vi "Test Write Speed.vi"(8 "error in (no error)":errorcluster, 11 "Path":path) -> (0 "error out":errorcluster, 1 "sizes":T2, 2 "Write Times":T1)   [LabVIEW 2016]
uses:
  Data.ITX/Data.ITX.lvclass
  Data/Data.lvclass
  Data/Typedefs/Dictionary--cluster.ctl
  Data/Typedefs/File Type--enum.ctl
  C:/Users/patrick/Documents/GitHub/LV-to-ITX/src/Data/Data.lvclass
panel:
  out "State":string
  in  "OK":bool
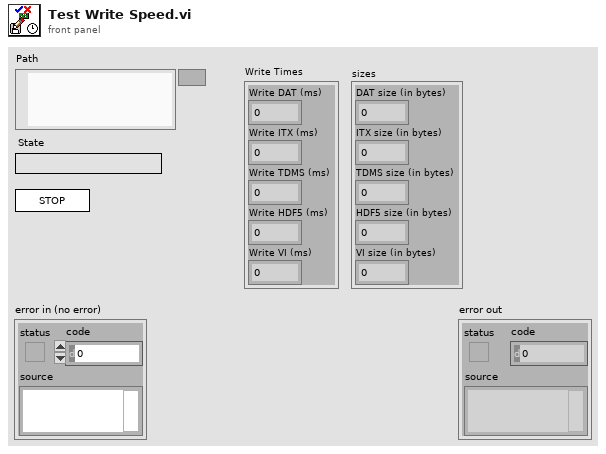
[diagram p1: front panel]
types:
  T1 = cluster{"Write DAT (ms)":u32, "Write ITX (ms)":u32, "Write TDMS (ms)":u32, "Write HDF5 (ms)":u32, "Write VI (ms)":u32}
  T2 = cluster{"DAT size (in bytes)":i64, "ITX size (in bytes)":i64, "TDMS size (in bytes)":i64, "HDF5 size (in bytes)":i64, "VI size (in bytes)":i64}
  T3 = enum32{"Invalid", "Standard", "Closed", "Hidden", "Minimized", "Maximized"}
  T4 = enum32{"invalid app kind", "Development System", "Run Time System", "Student Edition", "Embedded LabVIEW", "Evaluation", "Custom"}
  T5 = typedef "Data.lvclass/File Type--enum.ctl" = enum16{"DAT", "ITX", "TDMS", "VI"}
  T6 = typedef "Data.lvclass/Dictionary--cluster.ctl" = cluster{"key":string, "value":variant}
  T7 = cluster{"Core":cluster{"Current VI Reference":refnum<vi>, "Close Panel on Exit?":bool}, "Data (Dictionary)":T6[], "Path":path, "dat Path":path, "itx Path":path, "tdms Path":path, "hdf5 Path":path, "vi Path":path, "Write Times":cluster{"Write DAT (ms)":u32, "Write ITX (ms)":u32, "Write TDMS (ms)":u32, "Write HDF5 (ms)":u32, "Write VI (ms)":u32}, "Data Save out":refnum<class "Data.ITX.lvclass">}
  T8 = cluster{"Current VI Reference":refnum<vi>, "Close Panel on Exit?":bool}
  T9 = cluster{"size (in bytes)":i64, "size (in bytes)":i64, "size (in bytes)":i64, "size (in bytes)":i64, "size (in bytes)":i64}
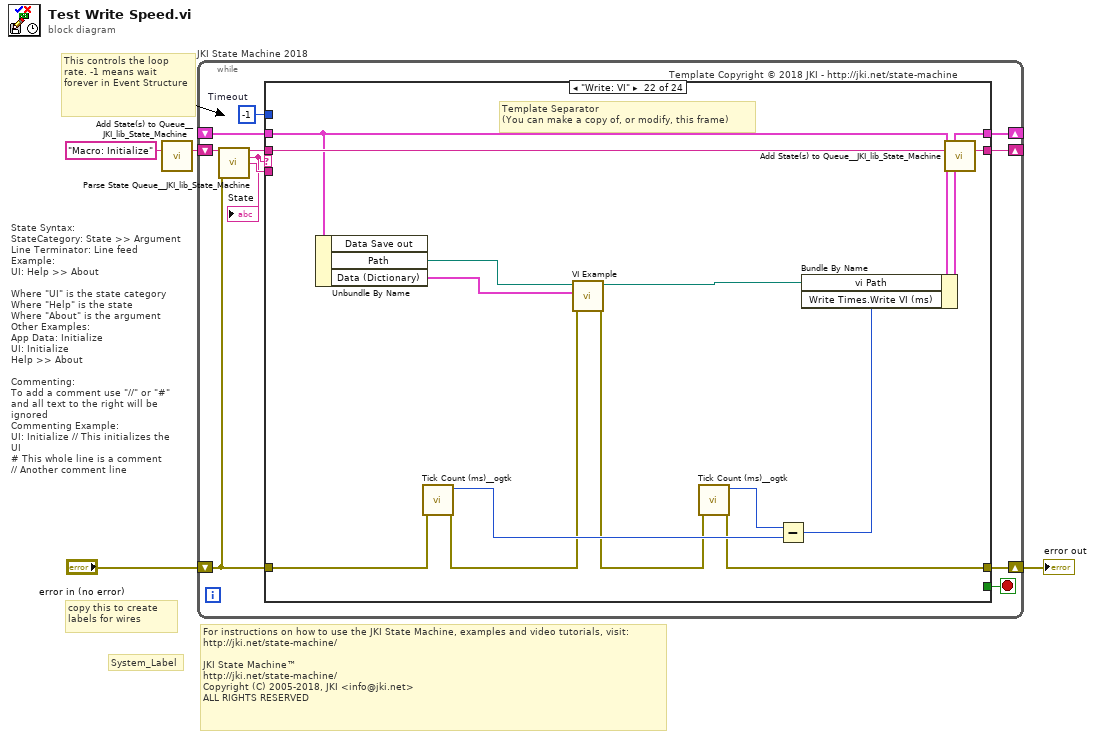
[diagram p0: block diagram]
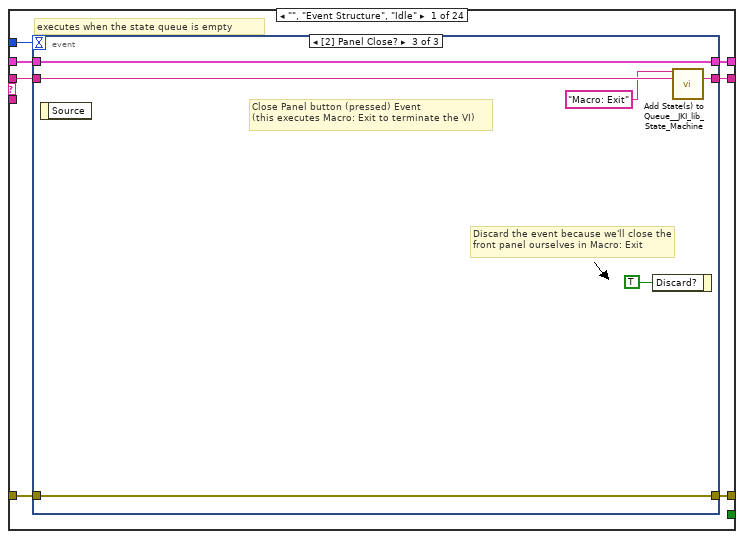
[diagram p2: hidden frame]
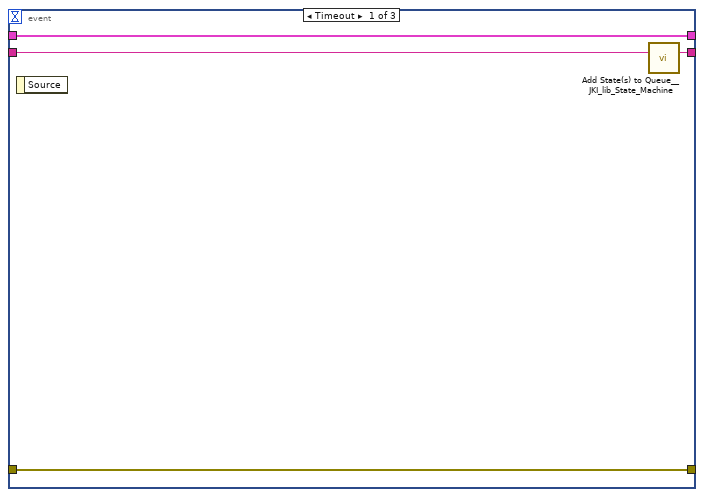
[diagram p3: hidden frame]
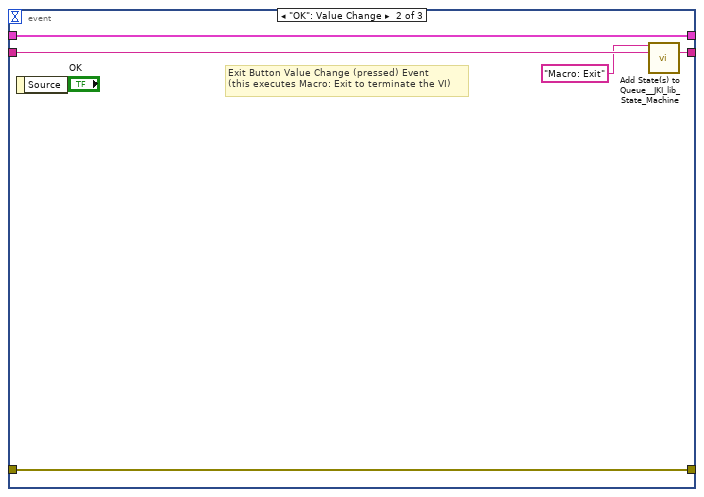
[diagram p4: hidden frame]
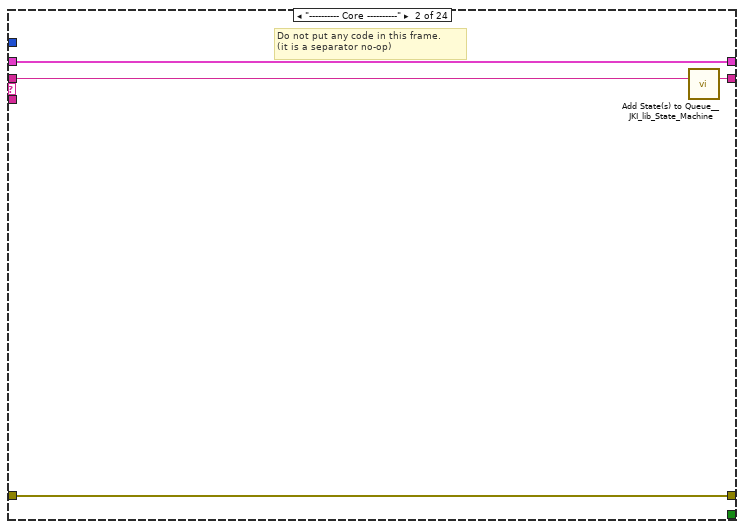
[diagram p5: hidden frame]
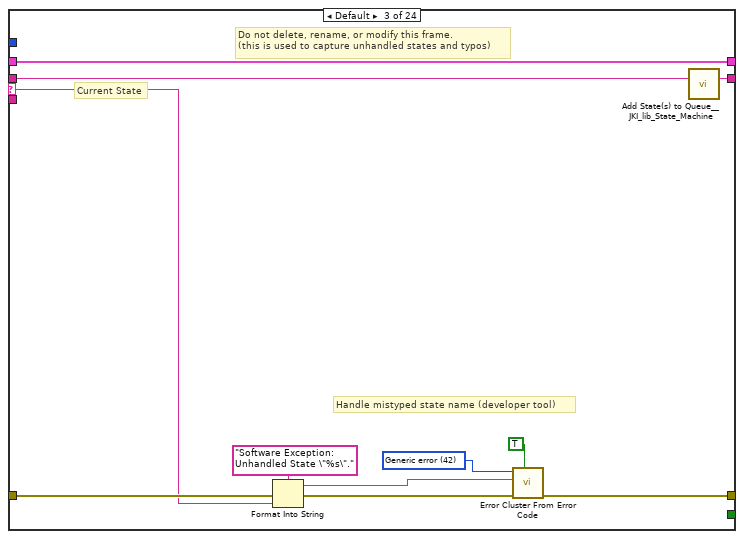
[diagram p6: hidden frame]
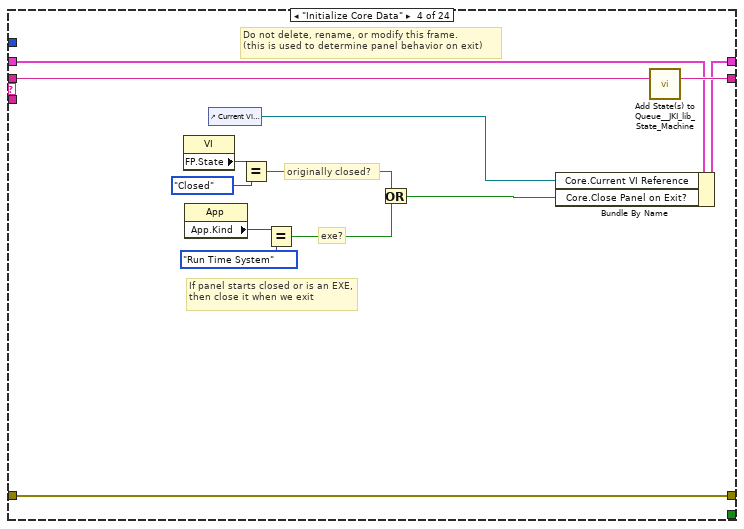
[diagram p7: hidden frame]
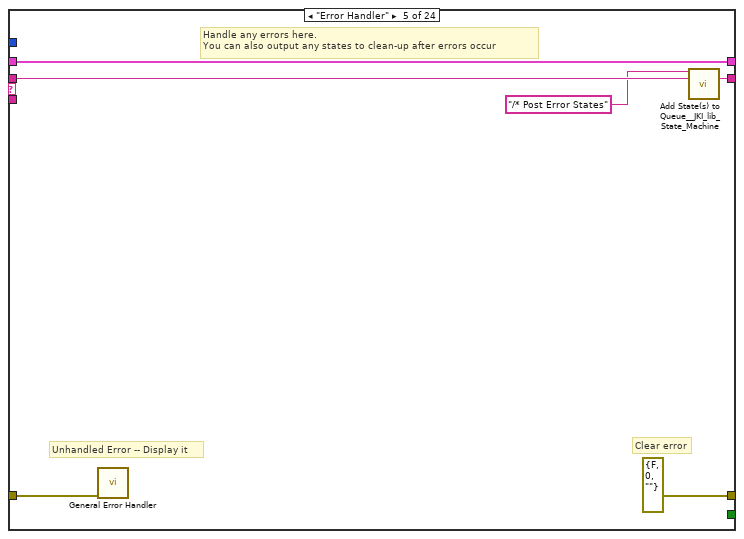
[diagram p8: hidden frame]
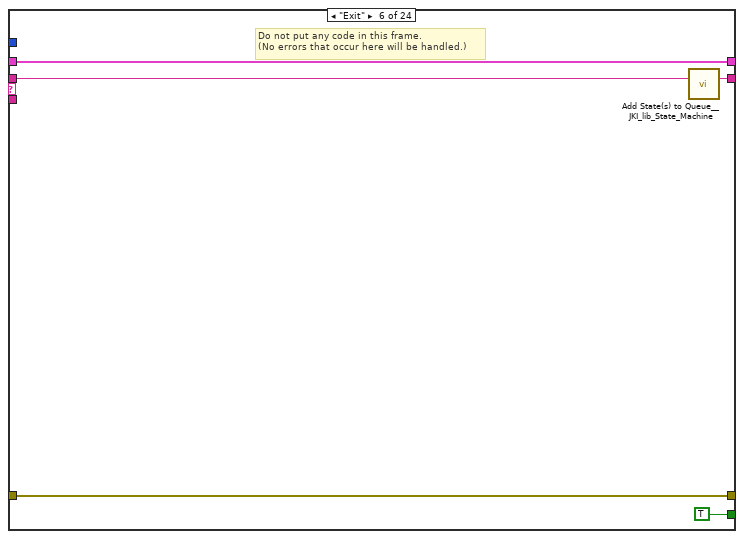
[diagram p9: hidden frame]
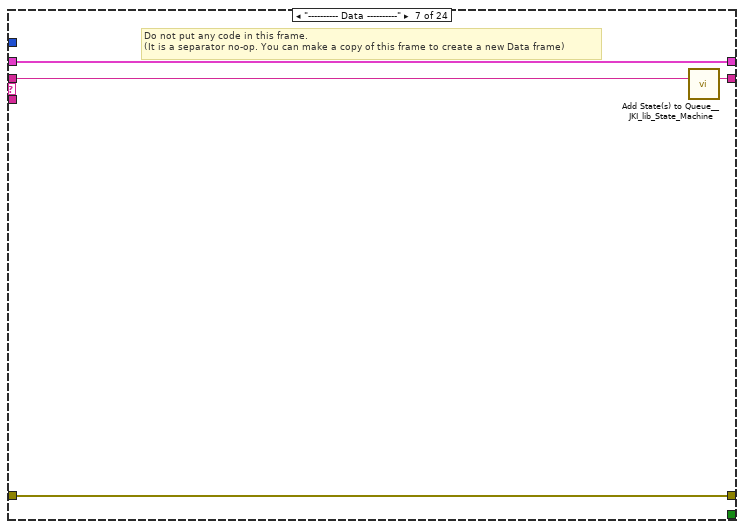
[diagram p10: hidden frame]
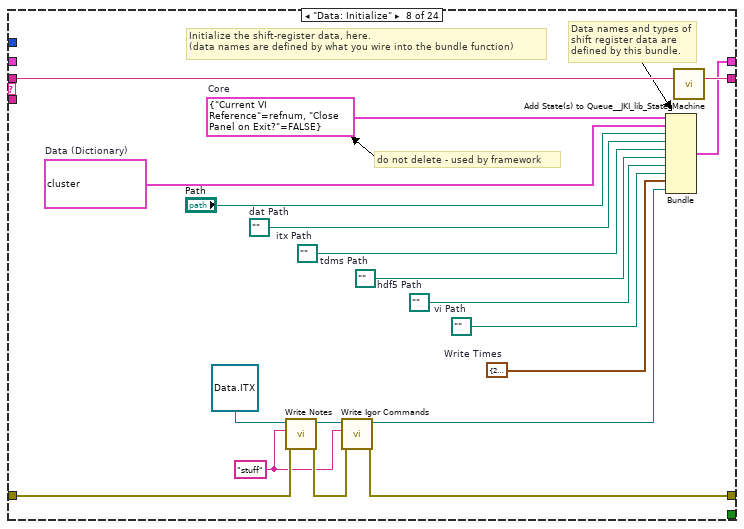
[diagram p11: hidden frame]
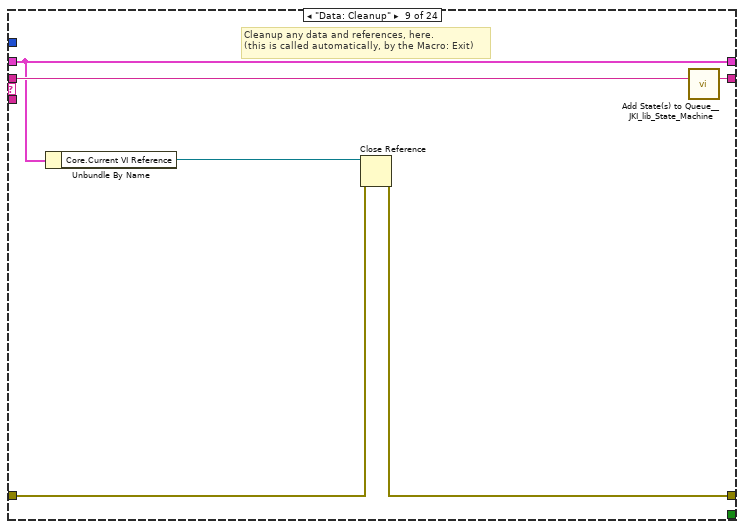
[diagram p12: hidden frame]
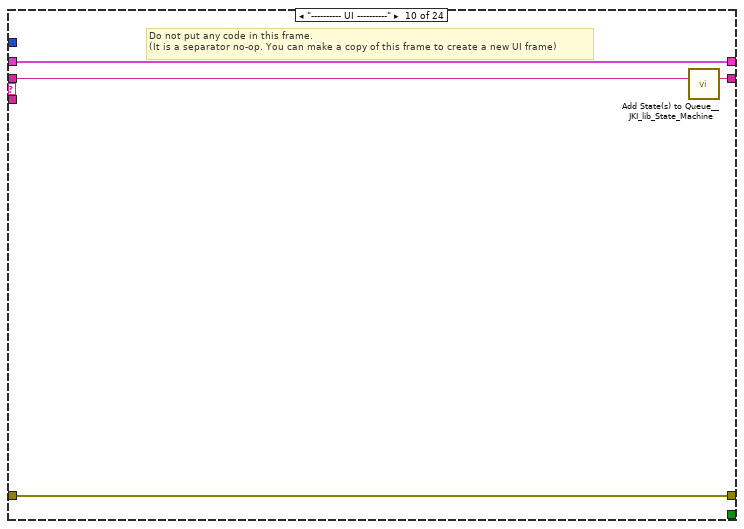
[diagram p13: hidden frame]
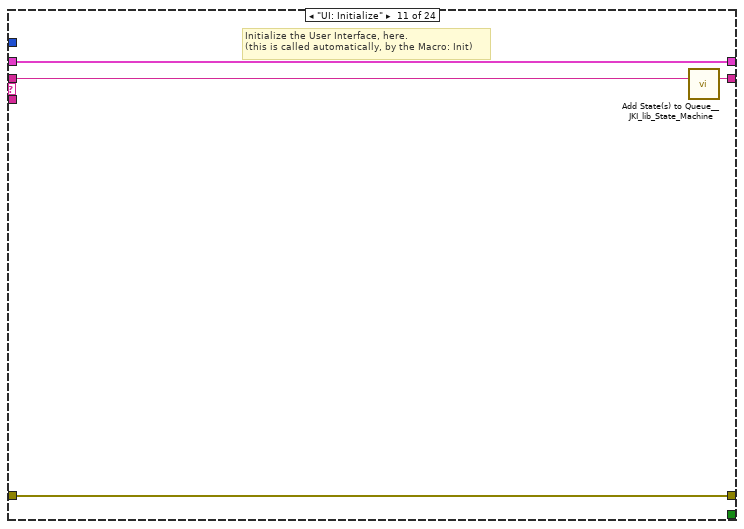
[diagram p14: hidden frame]
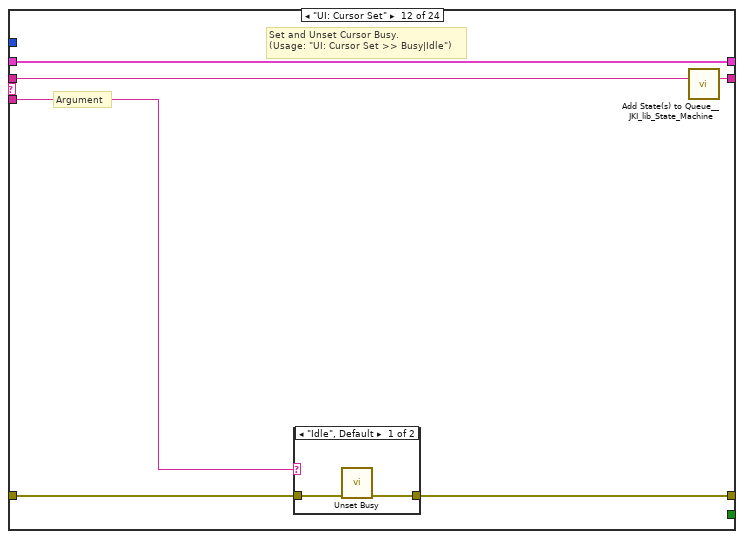
[diagram p15: hidden frame]
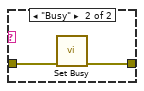
[diagram p16: hidden frame]
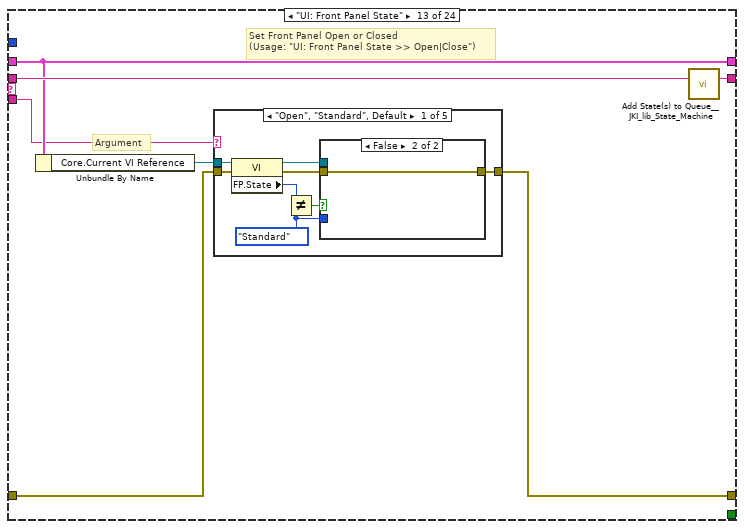
[diagram p17: hidden frame]
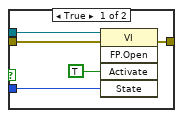
[diagram p18: hidden frame]
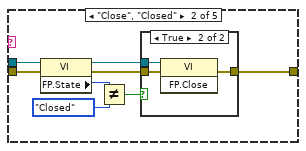
[diagram p19: hidden frame]
diagram:
  # "For instructions on how to use the JKI State Machine, examples and video tutorials, visit:\nhttp://jki.net/state-machine/\n\nJKI State Machine™\nhttp://jki.net/state-machine/\nCopyright (C) 2005-2018, JKI <info@jki.net>\nALL RIGHTS RESERVED"
  # "State Syntax:\nStateCategory: State >> Argument\nLine Terminator: Line feed\nExample:\nUI: Help >> About\n\nWhere \"UI\" is the state category\nWhere \"Help\" is the state\nWhere \"About\" is the argument\nOther Examples:\nApp Data: Initialize\nUI: Initialize\nHelp >> About\n\nCommenting:\nTo add a comment use \"//\" or \"#\" and all text to the right will be ignored\nCommenting Example:\nUI: Initialize // This initializes the UI\n# This whole line is a comment\n// Another comment line"
  # "copy this to create labels for wires"
  # "This controls the loop rate. -1 means wait forever in Event Structure"
  # "System_Label"
  n1 = call <vilib>:"Add State(s) to Queue__JKI_lib_State_Machine.vi"("State(s) in (\"\")"="Macro: Initialize") -> ("States Out"=w4:string)  [unwired: 14 in]
  n2 = while "JKI State Machine 2018" {
    shift-right: [w9] -> _
    shift-left: _ -> [w8]
    shift-right: [w12] -> w1
    shift-left: "error in (no error)" -> [w6]
    shift-right: [w11] -> _
    shift-left: w4 -> [w13]
    stop <- w10 stop-if-true
    w7 = -1  # Timeout
    # "Template Copyright © 2018 JKI - http://jki.net/state-machine"
    n3 = call <vilib>:"Parse State Queue__JKI_lib_State_Machine.vi"("State Queue"=w13, "Error In (no error)"=w6) -> ("Remaining States"=w15:string, "Current State"=w5:string, "Arguments"=w14:string)  [unwired: 11 in]
    "State" <- w5
    n4 = case shown="\"Write: VI\"" w5 {
      selector: w5 -> [_ _ w42 _ _ _ _ _ _ _ _ _ _ _ _ _ _ _ _ _ _ _ _ _]
      tunnel: w15 -> [w22 w41 w46 w65 w71 w76 w80 w99 w105 w109 w113 w119 w130 w199 w204 w209 w219 w223 w241 w258 w275 w289 w310 w322]
      tunnel: w14 -> [_ _ _ _ _ _ _ _ _ _ _ w114 w124 _ _ _ _ _ _ _ _ _ _ _]
      tunnel: w8 -> [w20 w38 w44 w58 w68 w74 w77 _ w100 w106 w111 w117 w126 w196 w201 w206 w216 w220 w236 w254 w267 w283 w308 w320]
      tunnel: [w19 w39 w48 w62 errorcluster {"status"=FALSE, "code"=0, "source"=""} ("error out") w73 w78 w90 w101 w107 w110 w115 w127 w197 w202 w207 w217 w221 w239 w255 w270 w284 w297 w315] -> w12
      tunnel: w6 -> [w18 w39 w47 w62 w67 w73 w78 w91 w102 w107 w110 w116 w128 w197 w202 w207 w217 w221 w234 w250 w271 w285 w307 w318]
      tunnel: [w21 w40 w45 w64 w70 w75 w79 w98 w104 w108 w112 w118 w129 w198 w203 w208 w218 w222 w240 w257 w274 w288 w309 w321] -> w11
      tunnel: [_ _ _ _ _ TRUE _ _ _ _ _ _ _ _ _ _ _ _ _ _ _ _ _ _] -> w10
      tunnel: [w17 w38 w44 w63 w68 w74 w77 w97 w100 w106 w111 w117 w126 w196 w201 w206 w216 w220 w235 w253 w266 w282 w308 w320] -> w9
      tunnel: w7 -> [w16 _ _ _ _ _ _ _ _ _ _ _ _ _ _ _ _ _ _ _ _ _ _ _]
      frame "", "Event Structure", "Idle" {
        # "executes when the state queue is empty"
        n5 = event shown="[2] Panel Close?" {
          selector: _ -> [_ _ _]
          dyn-events: _ -> [_ _ _]
          timeout: w16 -> [_ _ _]
          tunnel: w22 -> [w26 w31 w37]
          tunnel: [w25 w30 w36] -> w21
          tunnel: w20 -> [w23 w28 w34]
          tunnel: [w24 w29 w35] -> w19
          tunnel: w18 -> [w24 w29 w35]
          tunnel: [w23 w28 w34] -> w17
          event Timeout {
            n6 = event-data() -> ()  [unwired: 1 in, 1 out]
            n7 = call <vilib>:"Add State(s) to Queue__JKI_lib_State_Machine.vi"("State(s) in (\"\")"=w26) -> ("States Out"=w25:string)  [unwired: 14 in]
          }
          event "OK": Value Change {
            # "Exit Button Value Change (pressed) Event\n(this executes Macro: Exit to terminate the VI)"
            n8 = event-data() -> ()  [unwired: 1 in, 1 out]
            n9 = call <vilib>:"Add State(s) to Queue__JKI_lib_State_Machine.vi"("State(s) in Front (\"\")"="Macro: Exit", "State(s) in (\"\")"=w31) -> ("States Out"=w30:string)  [unwired: 13 in]
          }
          event Panel Close? {
            # "Discard the event because we'll close the front panel ourselves in Macro: Exit"
            # "Close Panel button (pressed) Event\n(this executes Macro: Exit to terminate the VI)"
            n10 = event-data() -> ()  [unwired: 1 in, 1 out]
            n11 = event-data("Discard?"=TRUE) -> ()  [unwired: 1 in, 1 out]
            n12 = call <vilib>:"Add State(s) to Queue__JKI_lib_State_Machine.vi"("State(s) in Front (\"\")"="Macro: Exit", "State(s) in (\"\")"=w37) -> ("States Out"=w36:string)  [unwired: 13 in]
          }
        }
      }
      frame "---------- Core ----------" {
        # "Do not put any code in this frame.\n(it is a separator no-op)"
        n13 = call <vilib>:"Add State(s) to Queue__JKI_lib_State_Machine.vi"("State(s) in (\"\")"=w41) -> ("States Out"=w40:string)  [unwired: 14 in]
      }
      frame Default {
        w51 = 42 items=["No error", "Argument error", "Memory is full", "Out of zone", "End of file", "File already open", "Generic file I/O error", "File not found", "File permission error", "Disk is full", "Duplicate path", "Too many files open", "System feature not enabled", "Resource file not found", "Cannot add resource", "Resource not found", "Image not found", "Image memory error", "Pen does not exist", "Config type invalid", "Config token not found", "Config parse error", "Config memory error", "Bad external code format", "Bad external code offset", "External code not present", "Null window", "Destroy window error", "Null menu", "Print aborted", "Bad print record", "Print driver error", "Windows error during printing", "Memory error during printing", "Print dialog error", "Generic print error", "Invalid device refnum", "Device not found", "Device parameter error", "Device unit error", "Cannot open device", "Device call aborted", "Generic error", "Cancelled by user", "Object ID too low", "Object ID too high", "Object not in heap", "Unknown heap", "Unknown object (invalid DefProc)", "Unknown object (DefProc not in table)", "Message out of range", "Invalid (null) method", "Unknown message", "Manager call not supported", "Bad address", "Network operation in progress", "Network operation timed out", "Connection is busy", "Network attribute not supported", "Network error", "Address in use", "System out of memory", "Connection aborted", "Connection refused", "Not connected", "Already connected", "Connection closed", "Initialization error (interapplication manager)", "Bad occurrence", "Wait on unbound occurrence handler", "Occurrence queue overflow", "Datalog type conflict", "Unused", "Unrecognized type (interapplication manager)", "Memory corrupt", "Failed to make temporary DLL", "Old CIN version", "Drag socket not found", "Failed to load drop-object", "Failed to register OLE object", "Failed to release OLE object", "Format specifier type mismatch", "Unknown format specifier", "Too few format specifiers", "Too many format specifiers", "Scan failed", "Newer CIN version", "Error converting to variant", "Runtime menu error", "Password tampered", "Variant attribute not found", "Incompatible variant data type", "Event data is not available", "Event Store is not present", "Occurrence is not found", "Event Queue is not created", "Event info is not available", "Refnum passed is NULL", "Error retrieving Class GUID", "Error retrieving CoClass GUID", "Error retrieving TypeLib GUID.", "Bad built application magic bytes.", "Specific driver is different from the specific driver associated with the Logical Name.", "There is no session opened to the class driver.", "Max Error", "MAX - Error with config objects", "MAX - Error loading configuration", "MAX - Group not supported"]
        # "Current State"
        # "Do not delete, rename, or modify this frame.\n(this is used to capture unhandled states and typos)"
        # "Handle mistyped state name (developer tool)"
        n14 = Format Into String(format string="Software Exception: Unhandled State \"%s\"." ("message"), error in=w47, w42) -> (resulting string=w50:string, error out=w49:errorcluster)  [unwired: 1 in]
        n15 = call <vilib>:"Error Cluster From Error Code.vi"("show call chain? (False)"=TRUE, "error in (no error)"=w49, "error message (\"\")"=w50, "error code (0)"=w51) -> ("error out"=w48:errorcluster)  [unwired: 5 in]
        n16 = call <vilib>:"Add State(s) to Queue__JKI_lib_State_Machine.vi"("State(s) in (\"\")"=w46) -> ("States Out"=w45:string)  [unwired: 14 in]
      }
      frame "Initialize Core Data" {
        # "Do not delete, rename, or modify this frame.\n(this is used to determine panel behavior on exit)"
        # "originally closed?"
        # "exe?"
        # "If panel starts closed or is an EXE, then close it when we exit"
        n17 = property class="VI"() -> ("FP.State"=w55:T3)  [unwired: 2 in, 2 out]
        n18 = property class="App"() -> ("App.Kind"=w61:T4)  [unwired: 2 in, 2 out]
        n19 = control-ref of="Current VI Reference"() -> (w56:refnum<vi>)
        n20 = Equal?(x=w55, y=T3."Closed" ("Front Panel Window:State")) -> (x = y?=w53:bool)
        n21 = Equal?(x=w61, y=T4."Run Time System" ("Application:Kind")) -> (x = y?=w59:bool)
        n22 = Or(x=w53, y=w59) -> (x .or. y?=w57:bool)
        n23 = Bundle By Name(cluster=w58, "Core.Current VI Reference"=w56, "Core.Close Panel on Exit?"=w57) -> (w63:T7)
        n24 = call <vilib>:"Add State(s) to Queue__JKI_lib_State_Machine.vi"("State(s) in (\"\")"=w65) -> ("States Out"=w64:string)  [unwired: 14 in]
      }
      frame "Error Handler" {
        # "Unhandled Error -- Display it"
        # "Handle any errors here.\nYou can also output any states to clean-up after errors occur"
        # "Clear error"
        n25 = call <vilib>:"General Error Handler.vi"("error in (no error)"=w67) -> ()  [unwired: 10 in, 5 out]
        n26 = call <vilib>:"Add State(s) to Queue__JKI_lib_State_Machine.vi"("State(s) in Front (\"\")"="/* Post Error States", "State(s) in (\"\")"=w71) -> ("States Out"=w70:string)  [unwired: 13 in]
      }
      frame "Exit" {
        # "Do not put any code in this frame.\n(No errors that occur here will be handled.)"
        n27 = call <vilib>:"Add State(s) to Queue__JKI_lib_State_Machine.vi"("State(s) in (\"\")"=w76) -> ("States Out"=w75:string)  [unwired: 14 in]
      }
      frame "---------- Data ----------" {
        # "Do not put any code in this frame.\n(It is a separator no-op. You can make a copy of this frame to create a new Data frame)"
        n28 = call <vilib>:"Add State(s) to Queue__JKI_lib_State_Machine.vi"("State(s) in (\"\")"=w80) -> ("States Out"=w79:string)  [unwired: 14 in]
      }
      frame "Data: Initialize" {
        w81 = T1 {"Write DAT (ms)"=2120, "Write ITX (ms)"=1952, "Write TDMS (ms)"=83, "Write HDF5 (ms)"=29, "Write VI (ms)"=2323}  # Write Times
        w82 = path ""  # vi Path
        w83 = T6[] [{"key"="time", "value"=variant(dbl[] array[87118 elements])}, {"key"="temp", "value"=variant(dbl[] array[87118 elements])}, {"key"="Bfield", "value"=variant(dbl[] array[87118 elements])}, {"key"="X0", "value"=variant(dbl[] array[87118 elements])}, {"key"="Y0", "value"=variant(dbl[] array[87118 elements])}, {"key"="X1", "value"=variant(dbl[] array[87118 elements])}, {"key"="Y1", "value"=variant(dbl[] array[87118 elements])}, {"key"="X2", "value"=variant(dbl[] array[87118 elements])}, {"key"="Y2", "value"=variant(dbl[] array[87118 elements])}, {"key"="X3", "value"=variant(dbl[] array[87118 elements])}, {"key"="Y3", "value"=variant(dbl[] array[87118 elements])}, {"key"="X4", "value"=variant(dbl[] array[87118 elements])}, {"key"="Y4", "value"=variant(dbl[] array[87118 elements])}, {"key"="X5", "value"=variant(dbl[] array[87118 elements])}, {"key"="Y5", "value"=variant(dbl[] array[87118 elements])}, {"key"="X6", "value"=variant(dbl[] array[87118 elements])}, {"key"="Y6", "value"=variant(dbl[] array[87118 elements])}, {"key"="X7", "value"=variant(dbl[] array[87118 elements])}, {"key"="Y7", "value"=variant(dbl[] array[87118 elements])}]  # Data (Dictionary)
        w84 = path ""  # hdf5 Path
        w85 = path ""  # tdms Path
        w86 = path ""  # itx Path
        w87 = path ""  # dat Path
        w88 = "stuff" ("Comments")
        w96 = T8 {"Current VI Reference"=refnum, "Close Panel on Exit?"=FALSE}  # Core
        # "do not delete - used by framework"
        # "Data names and types of shift register data are defined by this bundle."
        # "Initialize the shift-register data, here.\n(data names are defined by what you wire into the bundle function)"
        n29 = call "Write Notes.vi"("error in (no error)"=w91, "Notes"=w88, "Data Save"=refnum<class "Data.ITX.lvclass"> refnum ("LVtoITX in")) -> ("error out"=w89:errorcluster, "Data Save out"=w93:refnum<class "Data.ITX.lvclass">)  [unwired: 7 in]
        n30 = call "Write Igor Commands.vi"("error in (no error)"=w89, "Igor Commands"=w88, "Data Save"=w93) -> ("error out"=w90:errorcluster, "Data Save out"=w92:refnum<class "Data.ITX.lvclass">)  [unwired: 7 in]
        n31 = Bundle("Core"=w96, "Data (Dictionary)"=w83, "Path"="Path", "dat Path"=w87, "itx Path"=w86, "tdms Path"=w85, "hdf5 Path"=w84, "vi Path"=w82, "Write Times"=w81, "Data Save out"=w92) -> (w97:T7)  [unwired: 1 in]
        n32 = call <vilib>:"Add State(s) to Queue__JKI_lib_State_Machine.vi"("State(s) in (\"\")"=w99) -> ("States Out"=w98:string)  [unwired: 14 in]
      }
      frame "Data: Cleanup" {
        # "Cleanup any data and references, here.\n(this is called automatically, by the Macro: Exit)"
        n33 = Unbundle By Name(w100) -> ("Core.Current VI Reference"=w103:refnum<vi>)
        n34 = Close Reference(reference=w103, error in (no error)=w102) -> (error out=w101:errorcluster)
        n35 = call <vilib>:"Add State(s) to Queue__JKI_lib_State_Machine.vi"("State(s) in (\"\")"=w105) -> ("States Out"=w104:string)  [unwired: 14 in]
      }
      frame "---------- UI ----------" {
        # "Do not put any code in this frame.\n(It is a separator no-op. You can make a copy of this frame to create a new UI frame)"
        n36 = call <vilib>:"Add State(s) to Queue__JKI_lib_State_Machine.vi"("State(s) in (\"\")"=w109) -> ("States Out"=w108:string)  [unwired: 14 in]
      }
      frame "UI: Initialize" {
        # "Initialize the User Interface, here.\n(this is called automatically, by the Macro: Init)"
        n37 = call <vilib>:"Add State(s) to Queue__JKI_lib_State_Machine.vi"("State(s) in (\"\")"=w113) -> ("States Out"=w112:string)  [unwired: 14 in]
      }
      frame "UI: Cursor Set" {
        # "Argument"
        # "Set and Unset Cursor Busy.\n(Usage: \"UI: Cursor Set >> Busy|Idle\")"
        n38 = case shown="\"Idle\", Default" w114 {
          tunnel: w116 -> [w121 w123]
          tunnel: [w120 w122] -> w115
          frame "Idle", Default {
            n39 = call <vilib>:"Unset Busy.vi"("error in (no error)"=w121) -> ("error out"=w120:errorcluster)  [unwired: 10 in]
          }
          frame "Busy" {
            n40 = call <vilib>:"Set Busy.vi"("error in (no error)"=w123) -> ("error out"=w122:errorcluster)  [unwired: 9 in, 1 out]
          }
        }
        n41 = call <vilib>:"Add State(s) to Queue__JKI_lib_State_Machine.vi"("State(s) in (\"\")"=w119) -> ("States Out"=w118:string)  [unwired: 14 in]
      }
      frame "UI: Front Panel State" {
        # "Argument"
        # "Set Front Panel Open or Closed\n(Usage: \"UI: Front Panel State >> Open|Close\")"
        n42 = Unbundle By Name(w126) -> ("Core.Current VI Reference"=w125:refnum<vi>)
        n43 = case shown="\"Open\", \"Standard\", Default" w124 {
          tunnel: w128 -> [w136 w151 w162 w175 w188]
          tunnel: [w138 w152 w164 w177 w190] -> w127
          tunnel: w125 -> [w137 w149 w163 w176 w189]
          frame "Open", "Standard", Default {
            w131 = T3."Standard" ("State")
            n44 = property class="VI"(reference=w137, error in=w136) -> (reference out=w134:refnum<vi>, error out=w135:errorcluster, "FP.State"=w133:T3)
            n45 = Not Equal?(x=w133, y=w131) -> (x != y?=w132:bool)
            n46 = case shown="False" w132 {
              tunnel: [w142 w144] -> w138
              tunnel: w135 -> [w141 w144]
              tunnel: w134 -> [w140 _]
              tunnel: w131 -> [w139 _]
              frame True {
                n47 = invoke class="VI" method="FP.Open"(reference=w140, error in=w141, "Activate"=TRUE, "State"=w139) -> (error out=w142:errorcluster)  [unwired: 1 in, 4 out]
              }
              frame False {
              }
            }
          }
          frame "Close", "Closed" {
            n48 = property class="VI"(reference=w149, error in=w151) -> (reference out=w148:refnum<vi>, error out=w150:errorcluster, "FP.State"=w146:T3)
            n49 = Not Equal?(x=w146, y=T3."Closed" ("Front Panel Window:State")) -> (x != y?=w145:bool)
            n50 = case shown="True" w145 {
              tunnel: [w153 w156] -> w152
              tunnel: w150 -> [w153 w155]
              tunnel: w148 -> [_ w154]
              frame False {
              }
              frame True {
                n51 = invoke class="VI" method="FP.Close"(reference=w154, error in=w155) -> (error out=w156:errorcluster)  [unwired: 1 in, 2 out]
              }
            }
          }
          frame "Hidden", "Hide" {
            w157 = T3."Hidden" ("State")
            n52 = property class="VI"(reference=w163, error in=w162) -> (reference out=w160:refnum<vi>, error out=w161:errorcluster, "FP.State"=w159:T3)
            n53 = Not Equal?(x=w159, y=w157) -> (x != y?=w158:bool)
            n54 = case shown="True" w158 {
              tunnel: [w168 w169] -> w164
              tunnel: w161 -> [w167 w169]
              tunnel: w160 -> [w166 _]
              tunnel: w157 -> [w165 _]
              frame True {
                n55 = invoke class="VI" method="FP.Open"(reference=w166, error in=w167, "State"=w165) -> (error out=w168:errorcluster)  [unwired: 2 in, 4 out]
              }
              frame False {
              }
            }
          }
          frame "Minimize", "Minimized" {
            w170 = T3."Minimized" ("State")
            n56 = property class="VI"(reference=w176, error in=w175) -> (reference out=w173:refnum<vi>, error out=w174:errorcluster, "FP.State"=w172:T3)
            n57 = Not Equal?(x=w172, y=w170) -> (x != y?=w171:bool)
            n58 = case shown="True" w171 {
              tunnel: [w181 w182] -> w177
              tunnel: w174 -> [w180 w182]
              tunnel: w173 -> [w179 _]
              tunnel: w170 -> [w178 _]
              frame True {
                n59 = invoke class="VI" method="FP.Open"(reference=w179, error in=w180, "State"=w178) -> (error out=w181:errorcluster)  [unwired: 2 in, 4 out]
              }
              frame False {
              }
            }
          }
          frame "Maximize", "Maximized" {
            w183 = T3."Maximized" ("State")
            n60 = property class="VI"(reference=w189, error in=w188) -> (reference out=w186:refnum<vi>, error out=w187:errorcluster, "FP.State"=w185:T3)
            n61 = Not Equal?(x=w185, y=w183) -> (x != y?=w184:bool)
            n62 = case shown="True" w184 {
              tunnel: [w194 w195] -> w190
              tunnel: w187 -> [w193 w195]
              tunnel: w186 -> [w192 _]
              tunnel: w183 -> [w191 _]
              frame True {
                n63 = invoke class="VI" method="FP.Open"(reference=w192, error in=w193, "State"=w191) -> (error out=w194:errorcluster)  [unwired: 2 in, 4 out]
              }
              frame False {
              }
            }
          }
        }
        n64 = call <vilib>:"Add State(s) to Queue__JKI_lib_State_Machine.vi"("State(s) in (\"\")"=w130) -> ("States Out"=w129:string)  [unwired: 14 in]
      }
      frame "---------- Macro ----------" {
        # "Do not put any code in this frame.\n(It is a separator no-op. You can make a copy of this frame to create a new Macro frame)"
        n65 = call <vilib>:"Add State(s) to Queue__JKI_lib_State_Machine.vi"("State(s) in (\"\")"=w199) -> ("States Out"=w198:string)  [unwired: 14 in]
      }
      frame "Macro: Initialize" {
        # "Initialization Macro\n(This is called once, when the VI starts)"
        n66 = call <vilib>:"Add State(s) to Queue__JKI_lib_State_Machine.vi"("State(s) in Front (\"\")"="Data: Initialize\nInitialize Core Data\nUI: Initialize\nUI: Front Panel State >> Open\nMacro: Write", "State(s) in (\"\")"=w204) -> ("States Out"=w203:string)  [unwired: 13 in]
      }
      frame "Macro: Write" {
        # "Do not put any code in this frame.\n(It is a separator no-op. You can make a copy of this frame to create a new Macro frame)"
        n67 = call <vilib>:"Add State(s) to Queue__JKI_lib_State_Machine.vi"("State(s) in Front (\"\")"="Write: Cleanup\nWrite: DAT\nWrite: ITX\nWrite: TDMS\n//Write: VI\nWrite: Verify\nMacro: Exit", "State(s) in (\"\")"=w209) -> ("States Out"=w208:string)  [unwired: 13 in]
      }
      frame "Macro: Exit" {
        # "Exit Macro\n(This is called once, when the VI exits)"
        n68 = Unbundle By Name(w216) -> ("Core.Close Panel on Exit?"=w215:bool)
        n69 = Select(t="UI: Front Panel State >> Close", s=w215, f="") -> (s? t:f=w212:string)
        n70 = call <vilib>:"Add State(s) to Queue__JKI_lib_State_Machine.vi"("State(s) in (\"\")"=w212, "State(s) at Back (\"\")"="Data: Cleanup\nExit") -> ("States Out"=w210:string)  [unwired: 13 in]
        n71 = call <vilib>:"Add State(s) to Queue__JKI_lib_State_Machine.vi"("State(s) in Front (\"\")"=w210, "State(s) in (\"\")"=w219) -> ("States Out"=w218:string)  [unwired: 13 in]
      }
      frame "---------- Write ----------" {
        # "Template Separator\n(You can make a copy of, or modify, this frame)"
        n72 = call <vilib>:"Add State(s) to Queue__JKI_lib_State_Machine.vi"("State(s) in (\"\")"=w223) -> ("States Out"=w222:string)  [unwired: 14 in]
      }
      frame "Write: DAT" {
        # "Your code here.\n(You can make a copy of, or modify, this frame)"
        n73 = Unbundle By Name(w236) -> ("Path"=w229:path, "Data (Dictionary)"=w231:T6[])
        n74 = call <userlib>:"Tick Count (ms)__ogtk.vi"("error in (no error)"=w234) -> ("error out"=w230:errorcluster, "millisecond timer value"=w238:u32)  [unwired: 9 in]
        n75 = Build Path(base path=w229, name or relative path="filename" ("filename")) -> (appended path=w228:path)
        n76 = call "Data Write.vi"("File Type"=File_Type--enum."DAT", "Append Index"=0, "error in (no error)"=w230, "Data (Dictionary)"=w231, "path"=w228) -> ("error out"=w232:errorcluster, "path out"=w233:path)  [unwired: 5 in]
        n77 = call <userlib>:"Tick Count (ms)__ogtk.vi"("error in (no error)"=w232) -> ("error out"=w239:errorcluster, "millisecond timer value"=w237:u32)  [unwired: 9 in]
        n78 = Subtract(x=w237, y=w238) -> (x-y=w226:u32)
        n79 = Bundle By Name(cluster=w236, "dat Path"=w233, "Write Times.Write DAT (ms)"=w226) -> (w235:T7)
        n80 = call <vilib>:"Add State(s) to Queue__JKI_lib_State_Machine.vi"("State(s) in (\"\")"=w241) -> ("States Out"=w240:string)  [unwired: 14 in]
      }
      frame "Write: ITX" {
        # "Your code here.\n(You can make a copy of, or modify, this frame)"
        n81 = Unbundle By Name(w254) -> ("Path"=w251:path, "Data (Dictionary)"=w247:T6[])
        n82 = call <userlib>:"Tick Count (ms)__ogtk.vi"("error in (no error)"=w250) -> ("error out"=w246:errorcluster, "millisecond timer value"=w249:u32)  [unwired: 9 in]
        n83 = Build Path(base path=w251, name or relative path="filename" ("filename")) -> (appended path=w248:path)
        n84 = call "Data Write.vi"("File Type"=File_Type--enum."ITX", "error in (no error)"=w246, "Data (Dictionary)"=w247, "path"=w248) -> ("error out"=w245:errorcluster, "path out"=w244:path)  [unwired: 6 in]
        n85 = call <userlib>:"Tick Count (ms)__ogtk.vi"("error in (no error)"=w245) -> ("error out"=w255:errorcluster, "millisecond timer value"=w256:u32)  [unwired: 9 in]
        n86 = Subtract(x=w256, y=w249) -> (x-y=w243:u32)
        n87 = Bundle By Name(cluster=w254, "itx Path"=w244, "Write Times.Write ITX (ms)"=w243) -> (w253:T7)
        n88 = call <vilib>:"Add State(s) to Queue__JKI_lib_State_Machine.vi"("State(s) in (\"\")"=w258) -> ("States Out"=w257:string)  [unwired: 14 in]
      }
      frame "Write: TDMS" {
        # "Template Separator\n(You can make a copy of, or modify, this frame)"
        n89 = Unbundle By Name(w267) -> ("Path"=w269:path, "Data (Dictionary)"=w265:T6[])
        n90 = call <userlib>:"Tick Count (ms)__ogtk.vi"("error in (no error)"=w271) -> ("error out"=w263:errorcluster, "millisecond timer value"=w272:u32)  [unwired: 9 in]
        n91 = Build Path(base path=w269, name or relative path="filename") -> (appended path=w264:path)
        n92 = call "Data Write.vi"("File Type"=File_Type--enum."TDMS", "error in (no error)"=w263, "Data (Dictionary)"=w265, "path"=w264) -> ("error out"=w262:errorcluster, "path out"=w261:path)  [unwired: 6 in]
        n93 = call <userlib>:"Tick Count (ms)__ogtk.vi"("error in (no error)"=w262) -> ("error out"=w270:errorcluster, "millisecond timer value"=w273:u32)  [unwired: 9 in]
        n94 = Subtract(x=w273, y=w272) -> (x-y=w260:u32)
        n95 = Bundle By Name(cluster=w267, "tdms Path"=w261, "Write Times.Write TDMS (ms)"=w260) -> (w266:T7)
        n96 = call <vilib>:"Add State(s) to Queue__JKI_lib_State_Machine.vi"("State(s) in (\"\")"=w275) -> ("States Out"=w274:string)  [unwired: 14 in]
      }
      frame "Write: VI" {
        # "Template Separator\n(You can make a copy of, or modify, this frame)"
        n97 = Unbundle By Name(w283) -> ("Path"=w278:path, "Data (Dictionary)"=w279:T6[])  [unwired: 1 out]
        n98 = call <userlib>:"Tick Count (ms)__ogtk.vi"("error in (no error)"=w285) -> ("error out"=w281:errorcluster, "millisecond timer value"=w286:u32)  [unwired: 9 in]
        n99 = call "VI Example.vi"("error in (no error)"=w281, "Data (Dictionary)"=w279, "Path"=w278) -> ("error out"=w280:errorcluster, "saved file"=w277:path)  [unwired: 7 in]
        n100 = call <userlib>:"Tick Count (ms)__ogtk.vi"("error in (no error)"=w280) -> ("error out"=w284:errorcluster, "millisecond timer value"=w287:u32)  [unwired: 9 in]
        n101 = Subtract(x=w287, y=w286) -> (x-y=w276:u32)
        n102 = Bundle By Name(cluster=w283, "vi Path"=w277, "Write Times.Write VI (ms)"=w276) -> (w282:T7)
        n103 = call <vilib>:"Add State(s) to Queue__JKI_lib_State_Machine.vi"("State(s) in (\"\")"=w289) -> ("States Out"=w288:string)  [unwired: 14 in]
      }
      frame "Write: Verify" {
        # "Template Separator\n(You can make a copy of, or modify, this frame)"
        n104 = Unbundle By Name(w308) -> ("dat Path"=w303:path, "itx Path"=w302:path, "tdms Path"=w301:path, "hdf5 Path"=w300:path, "vi Path"=w299:path, "Write Times"=→"Write Times":T1)
        n105 = Get File Size(file=w303, error in=w307) -> (size (in bytes)=w296:i64, 0:w304:errorcluster)  [unwired: 1 out]
        n106 = Get File Size(file=w302, error in=w304) -> (size (in bytes)=w295:i64, 0:w305:errorcluster)  [unwired: 1 out]
        n107 = Get File Size(file=w301, error in=w305) -> (size (in bytes)=w292:i64, 0:w306:errorcluster)  [unwired: 1 out]
        n108 = Get File Size(file=w300, error in=w306) -> (size (in bytes)=w293:i64, 0:w298:errorcluster)  [unwired: 1 out]
        n109 = disable-structure shown="Disabled" {
          disable-tunnel: w299 -> [w314 _]
          disable-tunnel: w298 -> [w313 _]
          disable-tunnel: [w312 _] -> w297
          disable-tunnel: [w311 _] -> w294
          frame Disabled {
            n110 = Get File Size(file=w314, error in=w313) -> (size (in bytes)=w311:i64, 0:w312:errorcluster)  [unwired: 1 out]
          }
          frame Enabled {
          }
        }
        n111 = Bundle("size (in bytes)"=w296, "size (in bytes)"=w295, "size (in bytes)"=w292, "size (in bytes)"=w293, "size (in bytes)"=w294) -> (→"sizes":T9)  [unwired: 1 in]
        n112 = call <vilib>:"Add State(s) to Queue__JKI_lib_State_Machine.vi"("State(s) in (\"\")"=w310) -> ("States Out"=w309:string)  [unwired: 14 in]
      }
      frame "Write: Cleanup" {
        # "Template Separator\n(You can make a copy of, or modify, this frame)"
        n113 = Unbundle By Name(w320) -> ("Path"=w319:path)
        n114 = call <vilib>:"Recursive File List.vi"("error in (no error)"=w318, "Folder Path"=w319) -> ("error out"=w316:errorcluster, "All Files in Dir"=w317:path[])  [unwired: 5 in, 3 out]
        n115 = for {
          tunnel: w317 -> [w325] mode=indexing
          shift-right: [w323] -> w315
          shift-left: w316 -> [w324]
          n116 = Delete(path (use dialog)=w325, error in=w324) -> (error out=w323:errorcluster)  [unwired: 3 in, 2 out]
        }
        n117 = call <vilib>:"Add State(s) to Queue__JKI_lib_State_Machine.vi"("State(s) in (\"\")"=w322) -> ("States Out"=w321:string)  [unwired: 14 in]
      }
    }
  }
  "error out" <- w1
